vi "Get Queue Service Stats.vi"(8 "error in (no error)":errorcluster, 11 "Azure Session in":refnum<class "Session.lvclass">) -> (0 "error out":errorcluster, 1 "Last Sync Time":string, 2 "Status":string, 3 "Azure Session out":refnum<class "Session.lvclass">)   [LabVIEW 2015, in "NI_Azure_Queue.lvlib"]
doc: "Retrieves statistics related to replication for the Queue service."
uses:
  NI_Azure_Queue.lvlib
  Core/Session/Session.lvclass
  Core/Name Value Pair.ctl
  Core/Session/Session.lvclass/Session.ctl
  Core/Session/Write Request Parameters.vi
  Core/Session/Write HTTP Verb.vi
  Core/Session/Write _StorageAccountSuffix.vi
  Core/NI_Azure_Core.lvlib
  XML Parsing/NI_Azure_XML Parsing.lvlib
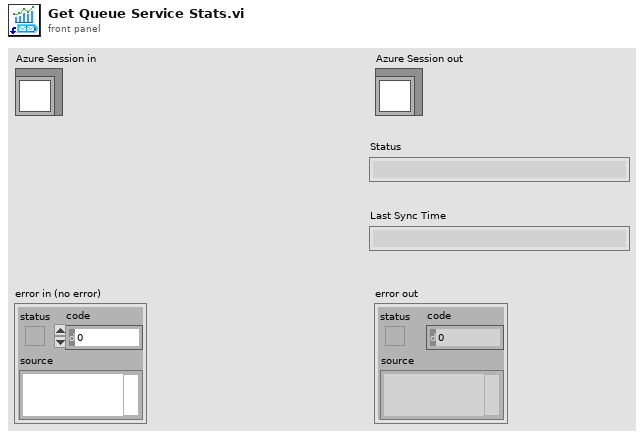
[diagram p1: front panel]
types:
  T1 = typedef "NI_Azure_Core.lvlib/Name Value Pair.ctl" = cluster{"name":string, "value":string}
  T2 = typedef "NI_Azure_Core.lvlib/Response.ctl" = cluster{"Headers":string, "Body":string}
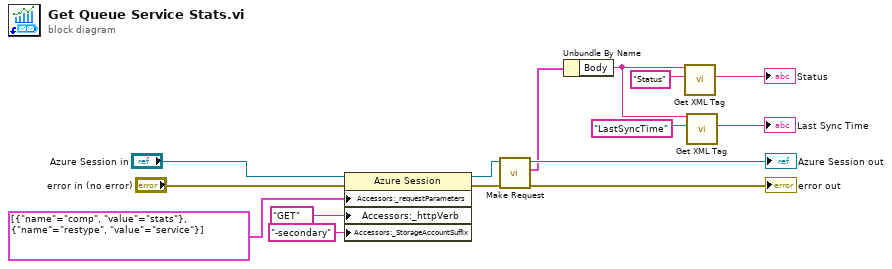
[diagram p0: block diagram]
diagram:
  n1 = property class="Azure Session"(reference="Azure Session in", error in="error in (no error)", "Accessors:_requestParameters"=T1[] [{"name"="comp", "value"="stats"}, {"name"="restype", "value"="service"}] ("request parameters"), "Accessors:_httpVerb"="GET" ("HTTP-Verb"), "Accessors:_StorageAccountSuffix"="-secondary" ("_StorageAccountSuffix")) -> (reference out=w9:refnum<class "Session.lvclass">, error out=w11:errorcluster)
  n2 = call "Make Request.vi"("error in (no error)"=w11, "Session in"=w9) -> ("error out"=→"error out":errorcluster, "Response"=w12:T2, "Session out"=→"Azure Session out":refnum<class "Session.lvclass">)  [unwired: 7 in]
  n3 = Unbundle By Name(w12) -> ("Body"=w3:string)
  n4 = call "Get XML Tag.vi"("Tag name"="Status", "XML String in"=w3) -> ("Tag value"=→"Status":string)  [unwired: 5 in, 4 out]
  n5 = call "Get XML Tag.vi"("Tag name"="LastSyncTime", "XML String in"=w3) -> ("Tag value"=→"Last Sync Time":string)  [unwired: 5 in, 4 out]
